vi "state_analysis.vi"(3 "current state number":dbl, 4 "postcharge state log file path":path, 5 "discharge state log file path":path, 6 "charge state log file path":path, 7 "predischarge state log file path":path) -> (0 "current state name":string, 1 "log? plot?":bool, 2 "chosen log file path":path)   [LabVIEW 2016]
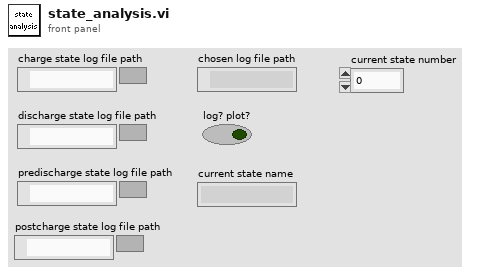
[diagram p1: front panel]
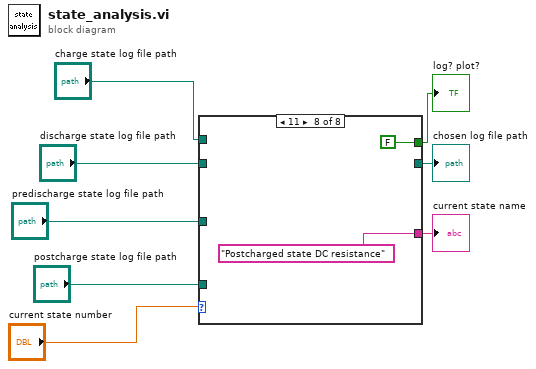
[diagram p0: block diagram]
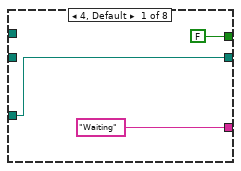
[diagram p2: hidden frame]
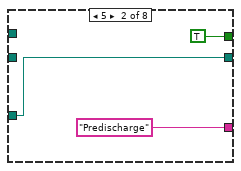
[diagram p3: hidden frame]
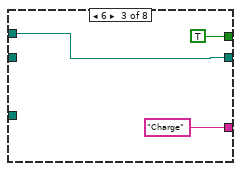
[diagram p4: hidden frame]
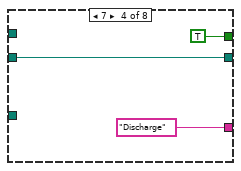
[diagram p5: hidden frame]
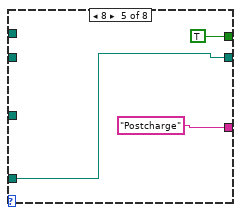
[diagram p6: hidden frame]
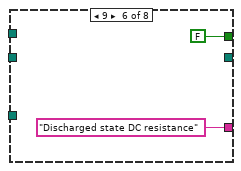
[diagram p7: hidden frame]
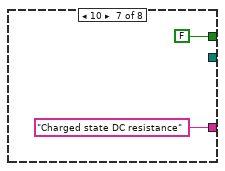
[diagram p8: hidden frame]
diagram:
  n1 = case shown="11" "current state number" {
    tunnel: "charge state log file path" -> [_ _ w15 _ _ _ _ _]
    tunnel: "discharge state log file path" -> [_ _ _ w18 _ _ _ _]
    tunnel: [w11 w14 w15 w18 w21 _ _ _] -> w6
    tunnel: "predischarge state log file path" -> [w11 w14 _ _ _ _ _ _]
    tunnel: ["Waiting" "Predischarge" "Charge" "Discharge" "Postcharge" "Discharged state DC resistance" "Charged state DC resistance" "Postcharged state DC resistance"] -> w5
    tunnel: [FALSE TRUE TRUE TRUE TRUE FALSE FALSE FALSE] -> w7
    tunnel: "postcharge state log file path" -> [_ _ _ _ w21 _ _ _]
    frame 4, Default {
    }
    frame 5 {
    }
    frame 6 {
    }
    frame 7 {
    }
    frame 8 {
    }
    frame 9 {
    }
    frame 10 {
    }
    frame 11 {
    }
  }
  "log? plot?" <- w7
  "chosen log file path" <- w6
  "current state name" <- w5
